vi "AddCrates.vi"(9 "To":i32, 10 "CratesToAdd":string[](array[string]), 11 "StacksIn":string[][](array[string])) -> (3 "StacksOut":string[][](array[string]))   [LabVIEW 2020, in "2022_5.lvclass"]
uses:
  2022_5.lvclass
  abd26ceb-1de9-4f31-8d3b-defafebb46df.vi
  abd26ceb-1de9-4f31-8d3b-defafebb46df.vi/be6f088c-3e4b-4523-ad48-2cdc85bad38a.vi
  abd26ceb-1de9-4f31-8d3b-defafebb46df.vi/f202eadf-433e-4cdb-b986-b2351ce8d73c.vi
  abd26ceb-1de9-4f31-8d3b-defafebb46df.vi/094751bc-bcf2-4346-afae-53942128b536.vi
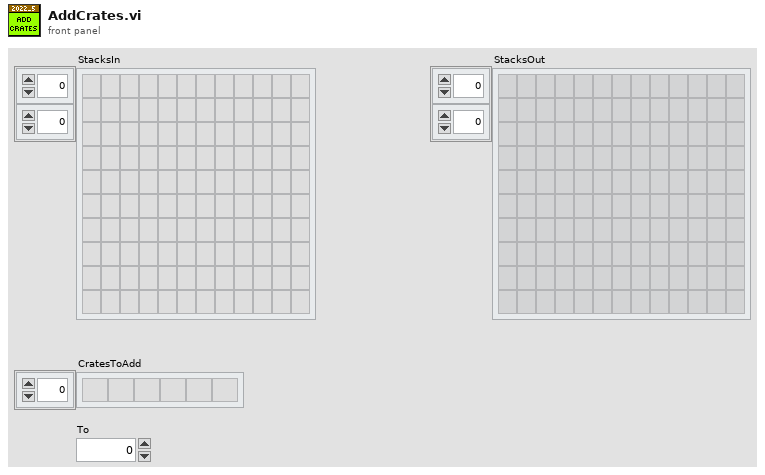
[diagram p1: front panel]
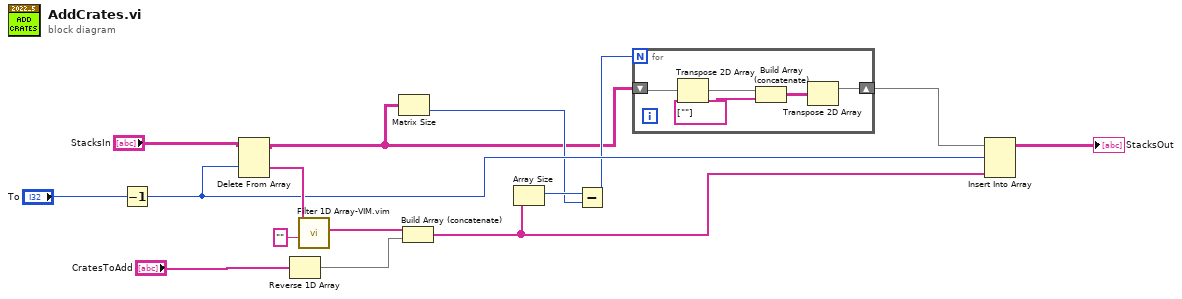
[diagram p0: block diagram]
diagram:
  n1 = Decrement(x="To") -> (x-1=w10:i32)
  n2 = Delete From Array(array="StacksIn", index (row)=w10) -> (deleted portion=w13:string[], array with subset deleted=w2:string[][])  [unwired: 2 in]
  n3 = Reverse 1D Array(array="CratesToAdd") -> (reversed array=w7:string[])
  n4 = call "Filter 1D Array-VIM.vim"("Item(s) to Filter"="", "Array"=w13) -> ("Filtered Array"=w9:string[])  [unwired: 5 in, 1 out]
  n5 = Matrix Size(0:w2) -> (2:w4:i32)  [unwired: 1 out]
  n6 = Build Array (concatenate)(w9, w7) -> (w6:string[])
  n7 = Array Size(array=w6) -> (size(s)=w5:i32)
  n8 = Subtract(x=w5, y=w4) -> (x-y=w3:i32)
  n9 = for {
    N: w3 -> [_]
    shift-right: [w16] -> w1
    shift-left: w2 -> [w20]
    n10 = Transpose 2D Array(2D array=w20) -> (transposed array=w19:string[][])
    n11 = Build Array (concatenate)(w19, string[] [""]) -> (w17:string[][])
    n12 = Transpose 2D Array(2D array=w17) -> (transposed array=w16:string[][])
  }
  n13 = Insert Into Array(array=w1, index (row)=w10, new element=w6) -> (→"StacksOut":string[][])  [unwired: 1 in]
